vi "My LevMar fit.vi"() -> ()   [LabVIEW 2016]
doc: "This demonstrates how to use nonlinear curve fitting to fit an ellipse. \nThis problem is modelled as a 2D curve fit (2 domains, 1 range), \nwhere the X and Y data are the noisy points, and Z is 1."
uses:
  <vilib>/gmath/NumericalOptimization/Nonlinear Curve Fit LM.vi
  <vilib>/gmath/NI_Gmath.lvlib
panel:
  in  "termination":cluster{"max iteration":i32, "tolerance":dbl}={"max iteration"=4000, "tolerance"=1e-08}
  out "Best Fit Parameters":dbl[](array[numeric])=[6.165966242609466, 0.5790994375004476, 1.1480005096376178, 1.5298484004229733, 0.19437479455605414, 0.3687918423691844, 0.42770434603605395, 0.2326334665057139, 0.05336680027829997] format="%_4g"
  in  "Input Parameters":dbl[](array[numeric])=[6.166, 0.5790850000000025, 1.148, 1.5297923499999972, 0.19443099999999983, 0.368831, 0.4277199999999989, 0.23264699999999988, 0.05337000000000001] format="%_4g"
  out "#function calls":i32=114
  out "residue":dbl=126.99491449057416
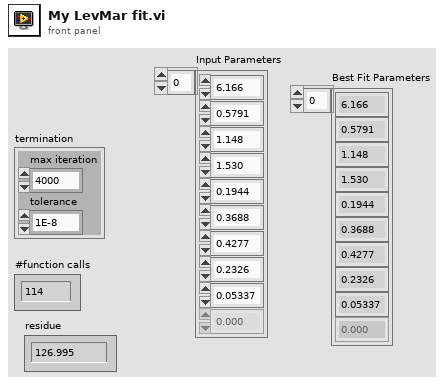
[diagram p1: front panel]
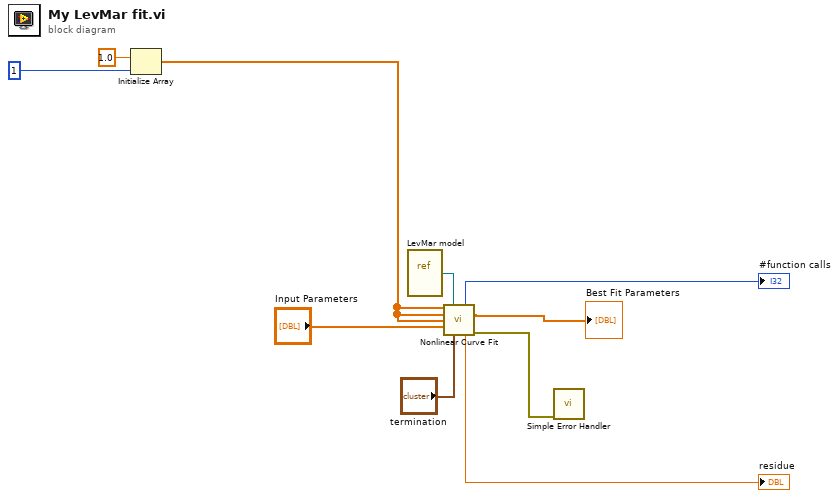
[diagram p0: block diagram]
diagram:
  n1 = Initialize Array(1.0, 1 ("samples")) -> (w3:dbl[])
  n2 = vi-ref "LevMar model.vi"() -> (w5:refnum<vi>)
  n3 = call-poly <vilib>:"Nonlinear Curve Fit.vi"("Y"=w3, "f(x,a)"=w5, "X"=w3, "Weight"=w3, "initial parameters"="Input Parameters", "termination"="termination") -> ("number of function calls"=→"#function calls":i32, "best fit parameters"=→"Best Fit Parameters":dbl[], "residue"=→"residue":dbl, "error out"=w4:errorcluster)  [unwired: 4 in, 2 out]
  n4 = call <vilib>:"Simple Error Handler.vi"("error in (no error)"=w4) -> ()  [unwired: 4 in, 5 out]
